vi "utilities_subtractTime.vi"(10 "number":dbl, 11 "Time":timestamp format="%<%X\n%x>T") -> (3 "Time out":timestamp format="%<%X\n%x>T")   [LabVIEW 2017, in "NI_ExcelFile.lvlib"]
uses:
  <vilib>/express/express shared/NI_ExcelFile/NI_ExcelFile.lvlib
  <vilib>/Utility/miscctls.llb/LVDateTimeRec.ctl
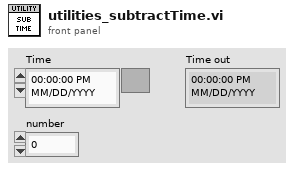
[diagram p1: front panel]
types:
  T1 = typedef "LVDateTimeRec.ctl" = cluster{"fractional second":dbl, "second":i32, "minute":i32, "hour":i32, "day of month":i32, "month":i32, "year":i32, "day of week":i32, "day of year":i32, "DST":i32}
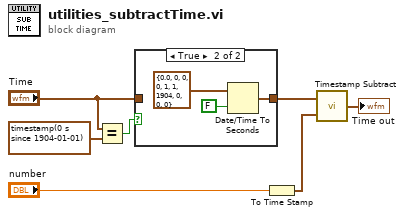
[diagram p0: block diagram]
diagram:
  n1 = Equal?(x="Time", y=timestamp(0 s since 1904-01-01)) -> (x = y?=w5:bool)
  n2 = case shown="True" w5 {
    tunnel: "Time" -> [w8 _]
    tunnel: [w8 w9] -> w3
    frame False {
    }
    frame True {
      n3 = Date/Time To Seconds(1:FALSE ("is UTC (F)"), 2:T1 {"fractional second"=0.0, "second"=0, "minute"=0, "hour"=0, "day of month"=1, "month"=1, "year"=1904, "day of week"=0, "day of year"=0, "DST"=0} ("date time rec")) -> (0:w9:timestamp)
    }
  }
  n4 = To Time Stamp(1:"number") -> (0:w2:timestamp)
  n5 = call <vilib>:"Timestamp Subtract.vi"("y"=w2, "x"=w3) -> ("x - y"=→"Time out":timestamp)
